vi "AutoSetUpMetodo.vi"(8 "error in (no error)":errorcluster, 11 "Keysight in":refnum<class "Keysight.lvclass">) -> (0 "error out":errorcluster, 3 "Keysight out":refnum<class "Keysight.lvclass">)   [LabVIEW 2020, in "Keysight.lvclass"]
uses:
  Keysight.lvclass
  Keysight.lvclass/Keysight.ctl
  <instrlib>/Agilent 2000 3000 X-Series/Agilent 2000 3000 X-Series.lvlib
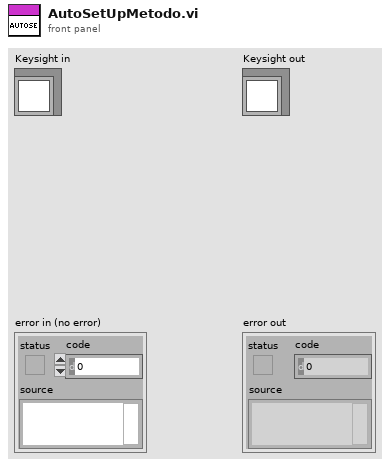
[diagram p1: front panel]
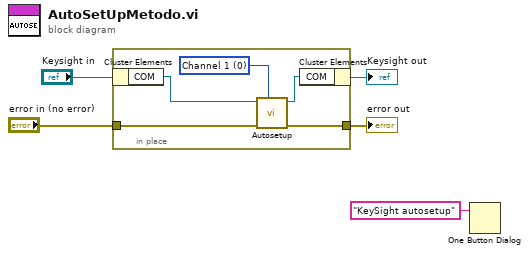
[diagram p0: block diagram]
diagram:
  n1 = in-place {
    in-place-border: "error in (no error)" -> [w8]
    in-place-border: [w7] -> w2
    w6 = 0 items=["Channel 1"=0, "Channel 2"=1, "Channel 3"=2, "Channel 4"=3, "Digital Bus Low"=9, "Digital Bus High"=10] ("Auto Scale Source (0: Channel 1)")
    n2 = in-place-cluster #1("Keysight in") -> ("COM"=w10:refnum<visa-resource-name>)
    n3 = call <instrlib>:"Autosetup.vi"("Auto Scale Source (0: Channel 1)"=w6, "error in (no error)"=w8, "VISA resource name"=w10) -> ("error out"=w7:errorcluster, "VISA resource name out"=w9:refnum<visa-resource-name>)  [unwired: 7 in]
    n4 = in-place-cluster #1("COM"=w9) -> (→"Keysight out":refnum<class "Keysight.lvclass">)
  }
  "error out" <- w2
  n5 = One Button Dialog(message="KeySight autosetup") -> ()  [unwired: 1 in, 1 out]
